vi "Write String.vi"(6 "error in (no error)":errorcluster, 7 "Bus In":refnum<class "Bus.lvclass">, 8 "Channel Name":string, 9 "Data Value Engineering":dbl, 10 "Data Value Native":dbl, 11 "No-Op in":refnum<class "No-Op Output.lvclass">) -> (0 "error out":errorcluster, 3 "No-Op out":refnum<class "No-Op Output.lvclass">, 5 "Bus Out":refnum<class "Bus.lvclass">)   [LabVIEW 2024, in "No-Op Output.lvclass"]
doc: "String Out.lvclass:Read String.vi\n\nThis is the template for the Read String VI forthe String Out class.\n\nInstrument Communication Module Version 1.0\nOctober, 2020 Original Code Consulting Davita Bird\n www.originalcode.com"
uses:
  No-Op Output.lvclass
  Bus/Bus.lvclass
  No-Op Output.lvclass/No-Op Output.ctl
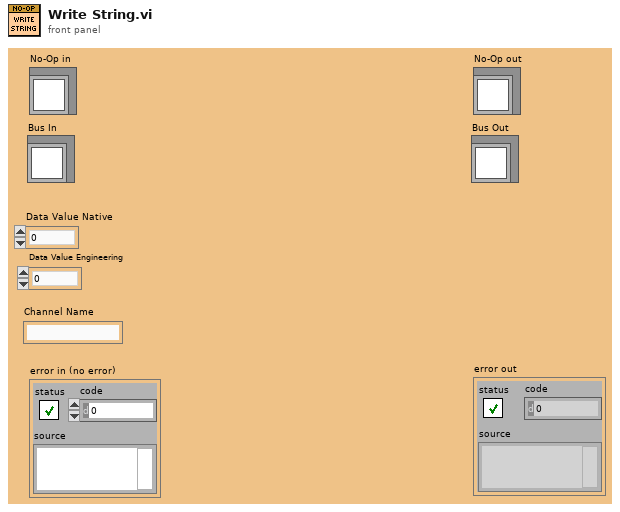
[diagram p1: front panel]
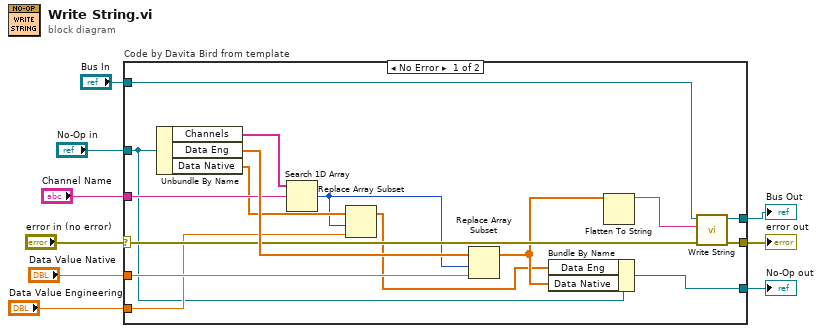
[diagram p0: block diagram]
diagram:
  n1 = case "Code by Davita Bird from template" shown="No Error" "error in (no error)" {
    selector: "error in (no error)" -> [w19 w28]
    tunnel: [w23 w28] -> w8
    tunnel: [w22 w27] -> w7
    tunnel: "No-Op in" -> [w11 w27]
    tunnel: "Data Value Native" -> [w20 _]
    tunnel: "Bus In" -> [w24 w26]
    tunnel: [w25 w26] -> w4
    tunnel: "Channel Name" -> [w16 _]
    tunnel: "Data Value Engineering" -> [w12 _]
    frame No Error {
      n2 = Unbundle By Name(w11) -> ("Channels"=w15:string[], "Data Eng"=w21:dbl[], "Data Native"=w14:dbl[])
      n3 = Search 1D Array(1D array=w15, element=w16) -> (index of element=w13:i32)  [unwired: 1 in]
      n4 = Replace Array Subset(array=w14, new element=w12, index=w13) -> (w10:dbl[])
      n5 = Replace Array Subset(array=w21, new element=w20, index=w13) -> (w17:dbl[])
      n6 = Bundle By Name(cluster=w11, "Data Eng"=w10, "Data Native"=w17) -> (w22:refnum<class "No-Op Output.lvclass">)
      n7 = Flatten To String(anything=w17) -> (data string=w18:string)  [unwired: 3 in, 2 out]
      n8 = call-dynamic "Write String.vi"("error in (no error)"=w19, "String"=w18, "Bus in"=w24) -> ("error out"=w23:errorcluster, "Bus out"=w25:refnum<class "Bus.lvclass">)  [unwired: 7 in]
    }
    frame Error {
    }
  }
  "error out" <- w8
  "No-Op out" <- w7
  "Bus Out" <- w4
